vi "Write TXT File.vi"(6 "Data Array":dbl[](array[numeric]), 8 "error in":errorcluster, 9 "Data & Time String":string, 10 "Header":string, 11 "Path":path) -> (0 "error out":errorcluster)   [LabVIEW 2011]
doc: "This subVI writes the object data to a file in a TXT format. \n\nAAL 9/09"
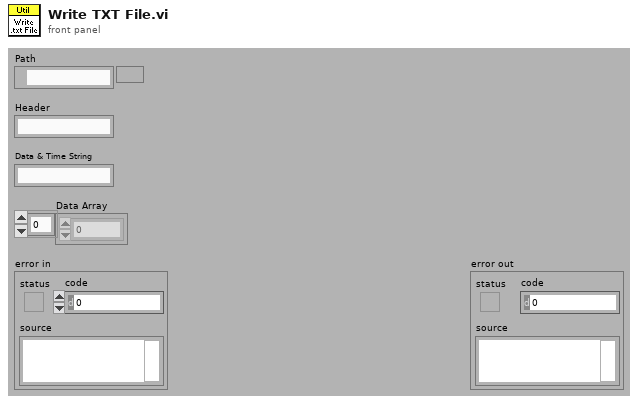
[diagram p1: front panel]
types:
  T1 = enum16{"open", "replace", "create", "open or create", "replace or create", "replace or create with confirmation"}
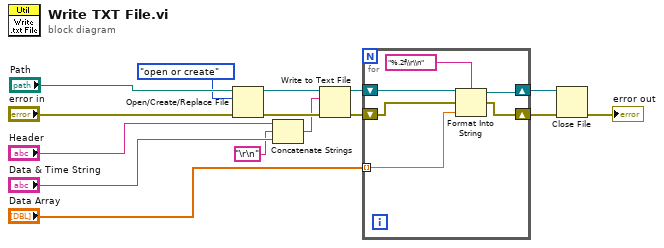
[diagram p0: block diagram]
diagram:
  n1 = Open/Create/Replace File(file path (use dialog)="Path", error in="error in", operation (0:open)=T1."open or create") -> (refnum out=w2:refnum<file>, error out=w5:errorcluster)  [unwired: 4 out]
  n2 = Concatenate Strings("Header", "\r\n", "Data & Time String") -> (w4:string)
  n3 = Write to Text File(file (use dialog)=w2, text=w4, error in=w5) -> (refnum out=w6:refnum<file>, error out=w7:errorcluster)  [unwired: 2 out]
  n4 = for {
    tunnel: "Data Array" -> [w21] mode=indexing
    shift-right: [w16] -> w9
    shift-left: w6 -> [w19]
    shift-right: [w17] -> w8
    shift-left: w7 -> [w18]
    n5 = Format Into String(format string="%.2f\\r\\n", initial string=w19, error in=w18, w21) -> (resulting string=w16:refnum<file>, error out=w17:errorcluster)
  }
  n6 = Close File(refnum=w9, error in=w8) -> (error out=→"error out":errorcluster)  [unwired: 1 out]
